vi "Configure Channel.vi"(8 "error in (no error)":errorcluster, 11 "Scope 1 Test in":refnum<class "Scope 1 Test.lvclass">) -> (0 "error out":errorcluster, 3 "Scope 1 Test out":refnum<class "Scope 1 Test.lvclass">)   [LabVIEW 2020, in "Oscilloscope VI.lvlib" / "Scope 1 Test.lvclass"]
uses:
  Scope 1 Test.lvclass
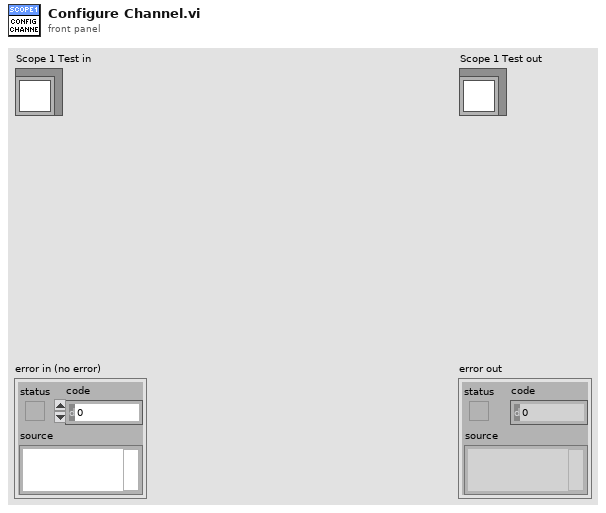
[diagram p1: front panel]
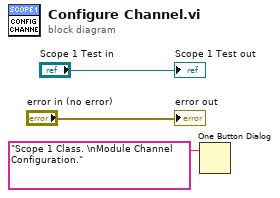
[diagram p0: block diagram]
diagram:
  n1 = One Button Dialog(message="Scope 1 Class. \nModule Channel Configuration.") -> ()  [unwired: 1 in, 1 out]
  "error out" <- "error in (no error)"
  "Scope 1 Test out" <- "Scope 1 Test in"
